vi "Get Timestamp.vi"(8 "error in":errorcluster, 11 "LogRecord in":refnum<class "LogRecord.lvclass">) -> (0 "error out":errorcluster, 2 "Created":timestamp, 3 "LogRecord out":refnum<class "LogRecord.lvclass">)   [LabVIEW 2024, in "hse-logger.lvlib" / "LogRecord.lvclass"]
doc: "Returns the timestamp of creating the LogRecord.\n\n____\nHAMPEL SOFTWARE ENGINEERING v2.2.2 (2025-01-16 15:41)"
uses:
  <vilib>/Hampel Software Engineering/HSE Logger/LogRecord/LogRecord.lvclass
  <vilib>/Hampel Software Engineering/HSE Logger/LogRecord/LogRecord.lvclass/LogRecord.ctl
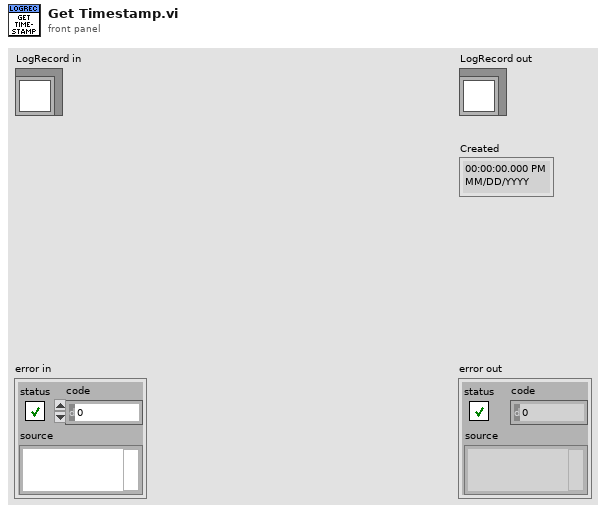
[diagram p1: front panel]
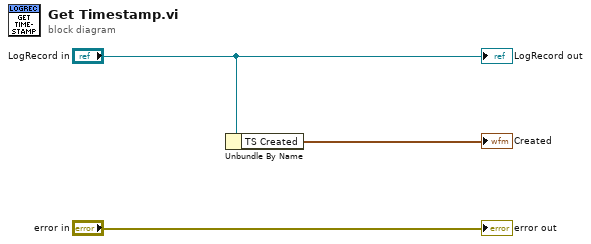
[diagram p0: block diagram]
diagram:
  n1 = Unbundle By Name("LogRecord in") -> ("TS Created"=→"Created":timestamp)
  "error out" <- "error in"
  "LogRecord out" <- "LogRecord in"
